vi "Write to Inline Execution Units.vi"(8 "error in (no error)":errorcluster, 11 "RTStateVariables in":T1 {"Inline Execution Units"."Outgoing Data References"."Data Reference" format="%.0x"; "Inline Execution Units"."Incoming Data References" format="%.0x"}) -> (0 "error out":errorcluster, 3 "RTStateVariables out":T1 {"Inline Execution Units"."Outgoing Data References"."Data Reference" format="%.0x"; "Inline Execution Units"."Incoming Data References" format="%.0x"})   [LabVIEW 2020, in "Communication Bus Template Engine.lvlib"]
uses:
  Communication Bus Template Engine.lvlib
  <vilib>/NI VeriStand/Custom Device API/Custom Device API.lvlib
  Includes/Communication Bus Engine.lvlibp/Interfaces/Execution Unit/Execution Unit.lvclass
  <vilib>/NI/NIVS Inline Async API/_VS Inline Async API/VS Inline Async API/VS Inline Async API.lvclass
  RTStateVariables.ctl
  <vilib>/NI VeriStand/Custom Device API/Data Reference.ctl
  <vilib>/NI VeriStand/Custom Device API/Block Data Reference.ctl
  Inline Execution Unit Runtime Information.ctl
  Asynchronous Execution Unit Runtime Information.ctl
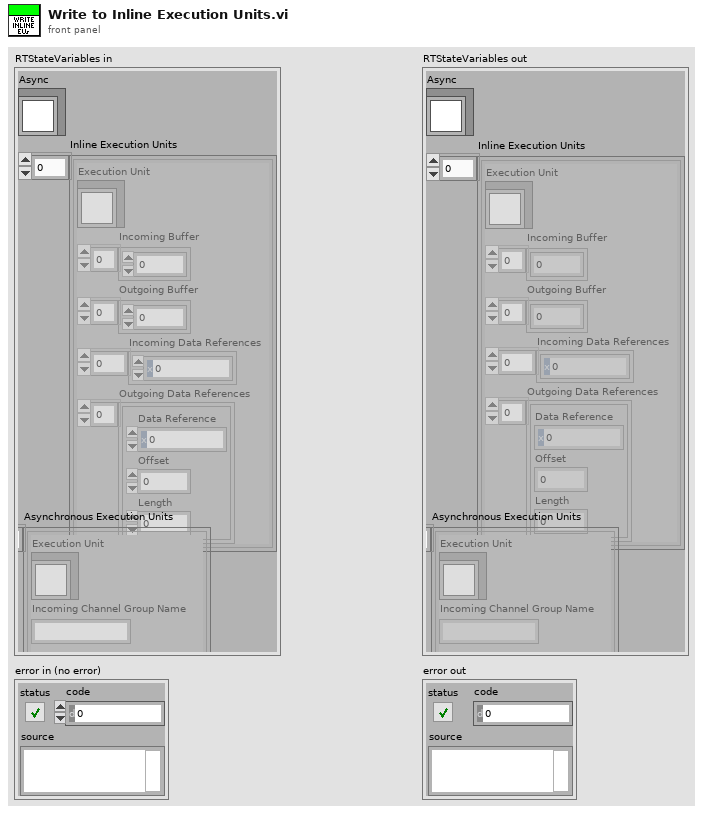
[diagram p1: front panel]
types:
  T1 = typedef "Communication Bus Template Engine.lvlib/RTStateVariables.ctl" = cluster{"Async":refnum<class "VS Inline Async API.lvclass">, "Inline Execution Units":T2[], "Asynchronous Execution Units":T5[]}
  T2 = typedef "Communication Bus Template Engine.lvlib/Inline Execution Unit Runtime Information.ctl" = cluster{"Execution Unit":refnum<class "Execution Unit.lvclass">, "Incoming Buffer":dbl[], "Outgoing Buffer":dbl[], "Incoming Data References":T3[], "Outgoing Data References":T4[]}
  T3 = typedef "Custom Device API.lvlib/Data Reference.ctl" = i32
  T4 = typedef "Custom Device API.lvlib/Block Data Reference.ctl" = cluster{"Data Reference":T3, "Offset":u64, "Length":u64}
  T5 = typedef "Communication Bus Template Engine.lvlib/Asynchronous Execution Unit Runtime Information.ctl" = cluster{"Execution Unit":refnum<class "Execution Unit.lvclass">, "Incoming Channel Group Name":string, "Outgoing Channel Group Name":string}
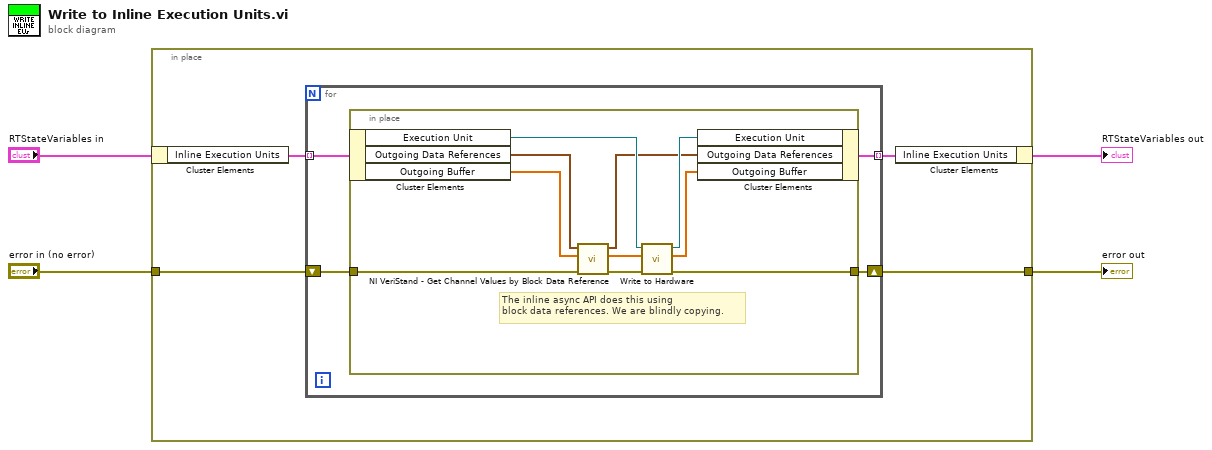
[diagram p0: block diagram]
diagram:
  n1 = in-place {
    in-place-border: [w8] -> w4
    in-place-border: "error in (no error)" -> [w7]
    n2 = in-place-cluster #1("RTStateVariables in") -> ("Inline Execution Units"=w6:T2[])
    n3 = for {
      tunnel: [w10] -> w5 mode=indexing
      tunnel: w6 -> [w9] mode=indexing
      shift-right: [w12] -> w8
      shift-left: w7 -> [w11]
      n4 = in-place {
        in-place-border: w11 -> [w18]
        in-place-border: [w19] -> w12
        # "The inline async API does this using\nblock data references. We are blindly copying."
        n5 = in-place-cluster #2(w9) -> ("Execution Unit"=w22:refnum<class "Execution Unit.lvclass">, "Outgoing Data References"=w14:T4[], "Outgoing Buffer"=w16:dbl[])
        n6 = call <vilib>:"NI VeriStand - Get Channel Values by Block Data Reference.vi"("error in (no error)"=w18, "Values Array in"=w16, "Block Data Ref"=w14) -> ("error out"=w17:errorcluster, "Values Array out"=w15:dbl[], "Block Data Ref dup"=w13:T4[])  [unwired: 6 in]
        n7 = call-dynamic "Write to Hardware.vi"("error in (no error)"=w17, "Values in"=w15, "Execution Unit in"=w22) -> ("error out"=w19:errorcluster, "Values out"=w20:dbl[], "Execution Unit out"=w21:refnum<class "Execution Unit.lvclass">)  [unwired: 6 in]
        n8 = in-place-cluster #2("Execution Unit"=w21, "Outgoing Data References"=w13, "Outgoing Buffer"=w20) -> (w10:T2)
      }
    }
    n9 = in-place-cluster #1("Inline Execution Units"=w5) -> (→"RTStateVariables out":T1)
  }
  "error out" <- w4
